vi "FPGA.Init.vi"(8 "error in (no error)":errorcluster) -> (0 "error out":errorcluster, 3 "Cluster":T1)   [LabVIEW 2015]
uses:
  Variables.ctl
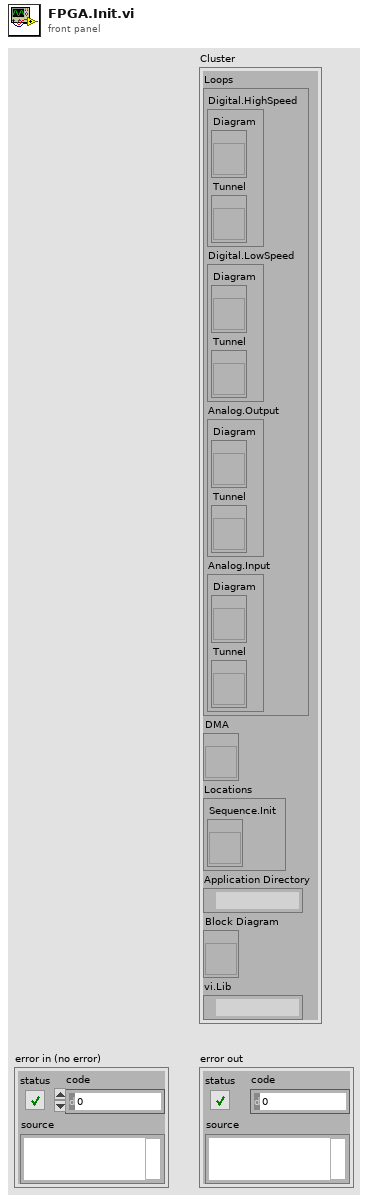
[diagram p1: front panel]
types:
  T1 = typedef "Variables.ctl" = cluster{"Loops":cluster{"Digital.HighSpeed":cluster{"Diagram":refnum<vi>, "Tunnel":refnum<vi>}, "Digital.LowSpeed":cluster{"Diagram":refnum<vi>, "Tunnel":refnum<vi>}, "Analog.Output":cluster{"Diagram":refnum<vi>, "Tunnel":refnum<vi>}, "Analog.Input":cluster{"Diagram":refnum<vi>, "Tunnel":refnum<vi>}}, "DMA":refnum<vi>, "Locations":cluster{"Sequence.Init":refnum<vi>}, "Application Directory":path, "Block Diagram":refnum<vi>, "vi.Lib":path}
  T2 = cluster{"Digital.HighSpeed":cluster{"Diagram":refnum<vi>, "Tunnel":refnum<vi>}, "Digital.LowSpeed":cluster{"Diagram":refnum<vi>, "Tunnel":refnum<vi>}, "Analog.Output":cluster{"Diagram":refnum<vi>, "Tunnel":refnum<vi>}, "Analog.Input":cluster{"Diagram":refnum<vi>, "Tunnel":refnum<vi>}}
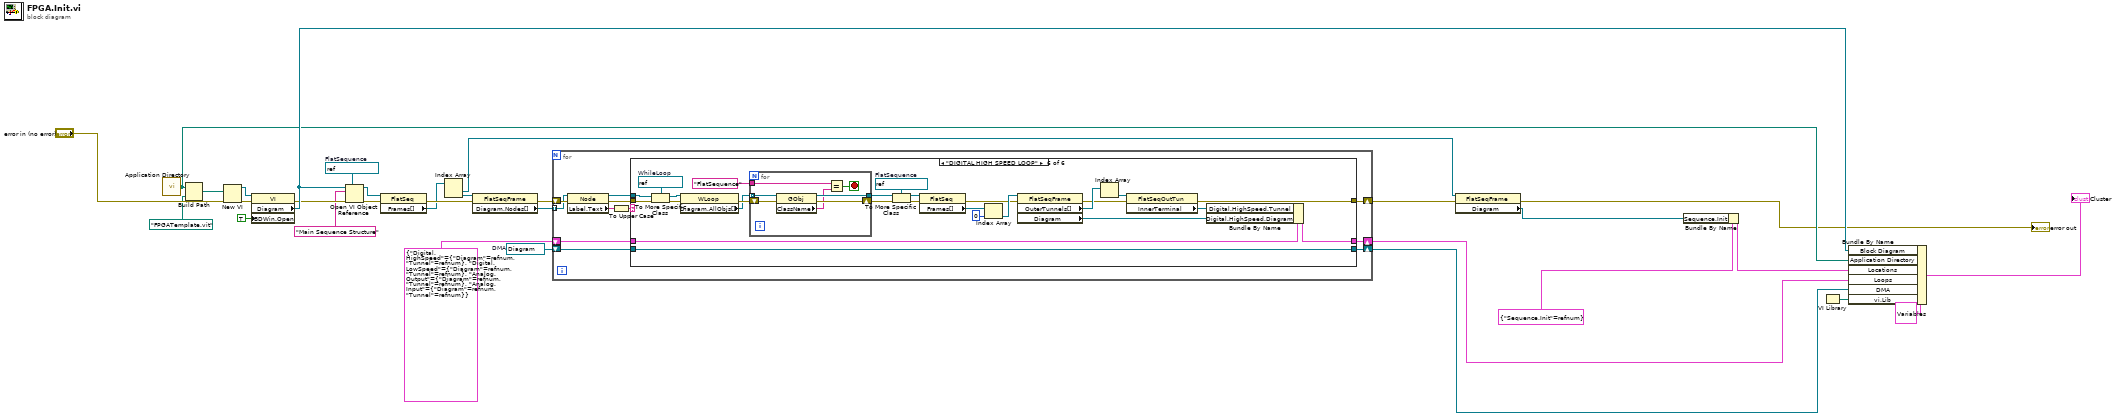
[diagram p0: block diagram]
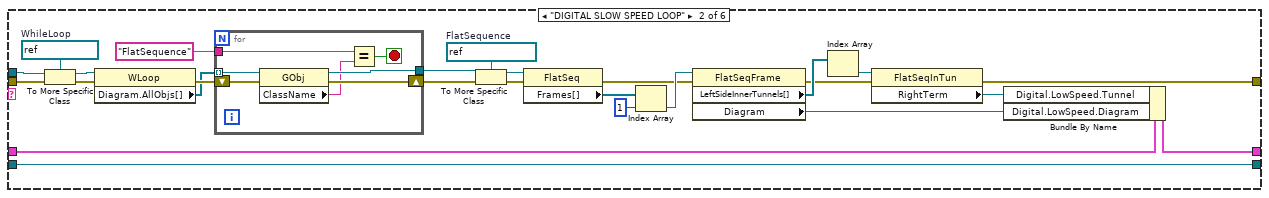
[diagram p3: hidden frame]
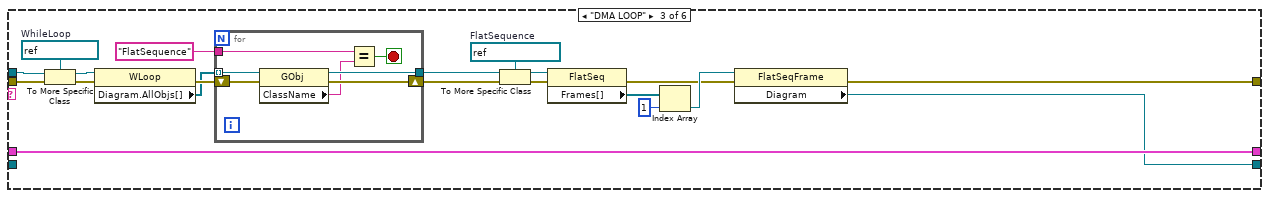
[diagram p4: hidden frame]
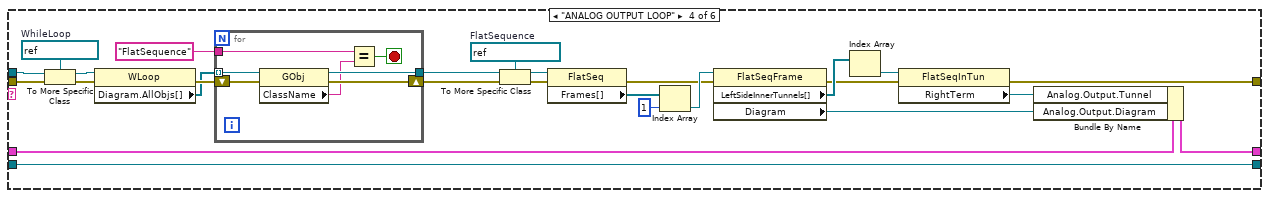
[diagram p5: hidden frame]
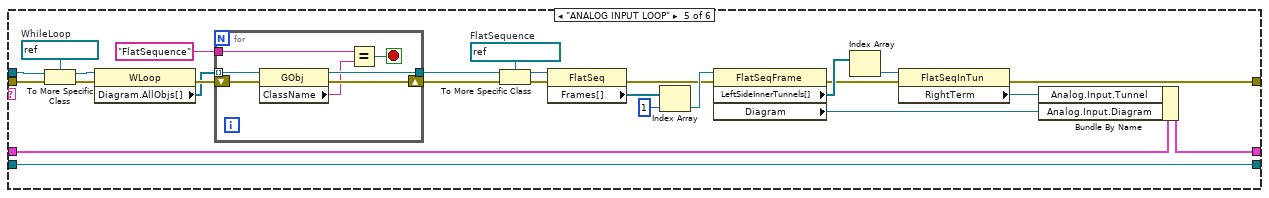
[diagram p6: hidden frame]
diagram:
  w17 = refnum<vi> refnum  # DMA
  w3 = refnum<vi> refnum  # FlatSequence
  n1 = call <vilib>:"Application Directory.vi"() -> ("Application Directory"=w28:path)
  n2 = Build Path(base path=w28, name or relative path=path "FPGATemplate.vit" ("template")) -> (appended path=w15:path)
  n3 = New VI(8:"error in (no error)", 10:w15) -> (0:w6:errorcluster, 3:w23:refnum<vi>)  [unwired: 5 in]
  n4 = property class="VI"(reference=w23, error in=w6, "BDWin.Open"=TRUE ("Block Diagram Window:Open")) -> (error out=w7:errorcluster, "Diagram"=w31:refnum<vi>)  [unwired: 1 out]
  n5 = Open VI Object Reference(7:w3, 8:w7, 10:"Main Sequence Structure" ("name/order"), 11:w31) -> (0:w9:errorcluster, 3:w8:refnum<vi>)
  n6 = property class="FlatSeq"(reference=w8, error in=w9) -> (error out=w11:errorcluster, "Frames[]"=w10:refnum<vi>[])  [unwired: 1 out]
  n7 = Index Array(array=w10) -> (element #1=w20:refnum<vi>, element #2=w18:refnum<vi>)  [unwired: 2 in]
  n8 = property class="FlatSeqFrame"(reference=w18, error in=w11) -> (error out=w13:errorcluster, "Diagram.Nodes[]"=w12:refnum<vi>[])  [unwired: 1 out]
  n9 = for {
    tunnel: w12 -> [w41] mode=indexing
    shift-right: [w35] -> w19
    shift-left: w13 -> [w42]
    shift-right: [w34] -> w27
    shift-left: T2 {"Digital.HighSpeed"={"Diagram"=refnum, "Tunnel"=refnum}, "Digital.LowSpeed"={"Diagram"=refnum, "Tunnel"=refnum}, "Analog.Output"={"Diagram"=refnum, "Tunnel"=refnum}, "Analog.Input"={"Diagram"=refnum, "Tunnel"=refnum}} -> [w38]
    shift-right: [w33] -> w30
    shift-left: w17 -> [w32]
    n10 = property class="Node"(reference=w41, error in=w42) -> (reference out=w37:refnum<vi>, error out=w36:errorcluster, "Label.Text"=w40:string)
    n11 = To Upper Case(1:w40) -> (0:w39:string)
    n12 = case shown="\"DIGITAL HIGH SPEED LOOP\"" w39 {
      tunnel: w38 -> [w44 w71 w80 w131 w164 w197]
      tunnel: w37 -> [_ w66 w95 w126 w159 w192]
      tunnel: w36 -> [w45 w67 w96 w127 w160 w193]
      tunnel: [w45 w48 w81 w107 w140 w173] -> w35
      tunnel: [w44 w70 w80 w130 w163 w196] -> w34
      tunnel: [w43 w52 w79 w112 w145 w178] -> w33
      tunnel: w32 -> [w43 w52 _ w112 w145 w178]
      frame Default {
      }
      frame "DIGITAL SLOW SPEED LOOP" {
        w65 = refnum<vi> refnum  # WhileLoop
        w58 = refnum<vi> refnum  # FlatSequence
        n13 = To More Specific Class(target class=w65, reference=w66, error in=w67) -> (specific class reference=w64:refnum<vi>, error out=w63:errorcluster)
        n14 = property class="WLoop"(reference=w64, error in=w63) -> (error out=w62:errorcluster, "Diagram.AllObjs[]"=w61:refnum<vi>[])  [unwired: 1 out]
        n15 = for {
          shift-right: [w77] -> w60
          shift-left: w62 -> [w78]
          tunnel: w61 -> [w76] mode=indexing
          tunnel: "FlatSequence" ("name/order") -> [w75]
          tunnel: [w73] -> w55
          stop <- w74 stop-if-true
          n16 = property class="GObj"(reference=w76, error in=w78) -> (reference out=w73:refnum<vi>, error out=w77:errorcluster, "ClassName"=w72:string)
          n17 = Equal?(x=w75, y=w72) -> (x = y?=w74:bool)
        }
        n18 = To More Specific Class(target class=w58, reference=w55, error in=w60) -> (specific class reference=w57:refnum<vi>, error out=w59:errorcluster)
        n19 = property class="FlatSeq"(reference=w57, error in=w59) -> (error out=w53:errorcluster, "Frames[]"=w69:refnum<vi>[])  [unwired: 1 out]
        n20 = Index Array(array=w69, index=1) -> (element=w54:refnum<vi>)
        n21 = property class="FlatSeqFrame"(reference=w54, error in=w53) -> (error out=w49:errorcluster, "LeftSideInnerTunnels[]"=w51:refnum<vi>[], "Diagram"=w46:refnum<vi>)  [unwired: 1 out]
        n22 = Index Array(array=w51) -> (element=w50:refnum<vi>)  [unwired: 1 in]
        n23 = property class="FlatSeqInTun"(reference=w50, error in=w49) -> (error out=w48:errorcluster, "RightTerm"=w47:refnum<vi>)  [unwired: 1 out]
        n24 = Bundle By Name(cluster=w71, "Digital.LowSpeed.Tunnel"=w47, "Digital.LowSpeed.Diagram"=w46) -> (w70:T2)
      }
      frame "DMA LOOP" {
        w94 = refnum<vi> refnum  # WhileLoop
        w87 = refnum<vi> refnum  # FlatSequence
        n25 = To More Specific Class(target class=w94, reference=w95, error in=w96) -> (specific class reference=w93:refnum<vi>, error out=w92:errorcluster)
        n26 = property class="WLoop"(reference=w93, error in=w92) -> (error out=w91:errorcluster, "Diagram.AllObjs[]"=w90:refnum<vi>[])  [unwired: 1 out]
        n27 = for {
          shift-right: [w104] -> w89
          shift-left: w91 -> [w105]
          tunnel: w90 -> [w103] mode=indexing
          tunnel: "FlatSequence" ("name/order") -> [w102]
          tunnel: [w100] -> w84
          stop <- w101 stop-if-true
          n28 = property class="GObj"(reference=w103, error in=w105) -> (reference out=w100:refnum<vi>, error out=w104:errorcluster, "ClassName"=w99:string)
          n29 = Equal?(x=w102, y=w99) -> (x = y?=w101:bool)
        }
        n30 = To More Specific Class(target class=w87, reference=w84, error in=w89) -> (specific class reference=w86:refnum<vi>, error out=w88:errorcluster)
        n31 = property class="FlatSeq"(reference=w86, error in=w88) -> (error out=w82:errorcluster, "Frames[]"=w98:refnum<vi>[])  [unwired: 1 out]
        n32 = Index Array(array=w98, index=1) -> (element=w83:refnum<vi>)
        n33 = property class="FlatSeqFrame"(reference=w83, error in=w82) -> (error out=w81:errorcluster, "Diagram"=w79:refnum<vi>)  [unwired: 1 out]
      }
      frame "ANALOG OUTPUT LOOP" {
        w125 = refnum<vi> refnum  # WhileLoop
        w118 = refnum<vi> refnum  # FlatSequence
        n34 = To More Specific Class(target class=w125, reference=w126, error in=w127) -> (specific class reference=w124:refnum<vi>, error out=w123:errorcluster)
        n35 = property class="WLoop"(reference=w124, error in=w123) -> (error out=w122:errorcluster, "Diagram.AllObjs[]"=w121:refnum<vi>[])  [unwired: 1 out]
        n36 = for {
          shift-right: [w137] -> w120
          shift-left: w122 -> [w138]
          tunnel: w121 -> [w136] mode=indexing
          tunnel: "FlatSequence" ("name/order") -> [w135]
          tunnel: [w133] -> w115
          stop <- w134 stop-if-true
          n37 = property class="GObj"(reference=w136, error in=w138) -> (reference out=w133:refnum<vi>, error out=w137:errorcluster, "ClassName"=w132:string)
          n38 = Equal?(x=w135, y=w132) -> (x = y?=w134:bool)
        }
        n39 = To More Specific Class(target class=w118, reference=w115, error in=w120) -> (specific class reference=w117:refnum<vi>, error out=w119:errorcluster)
        n40 = property class="FlatSeq"(reference=w117, error in=w119) -> (error out=w113:errorcluster, "Frames[]"=w129:refnum<vi>[])  [unwired: 1 out]
        n41 = Index Array(array=w129, index=1) -> (element=w114:refnum<vi>)
        n42 = property class="FlatSeqFrame"(reference=w114, error in=w113) -> (error out=w108:errorcluster, "LeftSideInnerTunnels[]"=w111:refnum<vi>[], "Diagram"=w106:refnum<vi>)  [unwired: 1 out]
        n43 = Index Array(array=w111) -> (element=w110:refnum<vi>)  [unwired: 1 in]
        n44 = property class="FlatSeqInTun"(reference=w110, error in=w108) -> (error out=w107:errorcluster, "RightTerm"=w109:refnum<vi>)  [unwired: 1 out]
        n45 = Bundle By Name(cluster=w131, "Analog.Output.Tunnel"=w109, "Analog.Output.Diagram"=w106) -> (w130:T2)
      }
      frame "ANALOG INPUT LOOP" {
        w158 = refnum<vi> refnum  # WhileLoop
        w151 = refnum<vi> refnum  # FlatSequence
        n46 = To More Specific Class(target class=w158, reference=w159, error in=w160) -> (specific class reference=w157:refnum<vi>, error out=w156:errorcluster)
        n47 = property class="WLoop"(reference=w157, error in=w156) -> (error out=w155:errorcluster, "Diagram.AllObjs[]"=w154:refnum<vi>[])  [unwired: 1 out]
        n48 = for {
          shift-right: [w170] -> w153
          shift-left: w155 -> [w171]
          tunnel: w154 -> [w169] mode=indexing
          tunnel: "FlatSequence" ("name/order") -> [w168]
          tunnel: [w166] -> w148
          stop <- w167 stop-if-true
          n49 = property class="GObj"(reference=w169, error in=w171) -> (reference out=w166:refnum<vi>, error out=w170:errorcluster, "ClassName"=w165:string)
          n50 = Equal?(x=w168, y=w165) -> (x = y?=w167:bool)
        }
        n51 = To More Specific Class(target class=w151, reference=w148, error in=w153) -> (specific class reference=w150:refnum<vi>, error out=w152:errorcluster)
        n52 = property class="FlatSeq"(reference=w150, error in=w152) -> (error out=w146:errorcluster, "Frames[]"=w162:refnum<vi>[])  [unwired: 1 out]
        n53 = Index Array(array=w162, index=1) -> (element=w147:refnum<vi>)
        n54 = property class="FlatSeqFrame"(reference=w147, error in=w146) -> (error out=w141:errorcluster, "LeftSideInnerTunnels[]"=w144:refnum<vi>[], "Diagram"=w139:refnum<vi>)  [unwired: 1 out]
        n55 = Index Array(array=w144) -> (element=w143:refnum<vi>)  [unwired: 1 in]
        n56 = property class="FlatSeqInTun"(reference=w143, error in=w141) -> (error out=w140:errorcluster, "RightTerm"=w142:refnum<vi>)  [unwired: 1 out]
        n57 = Bundle By Name(cluster=w164, "Analog.Input.Tunnel"=w142, "Analog.Input.Diagram"=w139) -> (w163:T2)
      }
      frame "DIGITAL HIGH SPEED LOOP" {
        w191 = refnum<vi> refnum  # WhileLoop
        w184 = refnum<vi> refnum  # FlatSequence
        n58 = To More Specific Class(target class=w191, reference=w192, error in=w193) -> (specific class reference=w190:refnum<vi>, error out=w189:errorcluster)
        n59 = property class="WLoop"(reference=w190, error in=w189) -> (error out=w188:errorcluster, "Diagram.AllObjs[]"=w187:refnum<vi>[])  [unwired: 1 out]
        n60 = for {
          shift-right: [w203] -> w186
          shift-left: w188 -> [w204]
          tunnel: w187 -> [w202] mode=indexing
          tunnel: "FlatSequence" ("name/order") -> [w201]
          tunnel: [w199] -> w181
          stop <- w200 stop-if-true
          n61 = property class="GObj"(reference=w202, error in=w204) -> (reference out=w199:refnum<vi>, error out=w203:errorcluster, "ClassName"=w198:string)
          n62 = Equal?(x=w201, y=w198) -> (x = y?=w200:bool)
        }
        n63 = To More Specific Class(target class=w184, reference=w181, error in=w186) -> (specific class reference=w183:refnum<vi>, error out=w185:errorcluster)
        n64 = property class="FlatSeq"(reference=w183, error in=w185) -> (error out=w179:errorcluster, "Frames[]"=w195:refnum<vi>[])  [unwired: 1 out]
        n65 = Index Array(array=w195, index=0) -> (element=w180:refnum<vi>)
        n66 = property class="FlatSeqFrame"(reference=w180, error in=w179) -> (error out=w174:errorcluster, "OuterTunnels[]"=w175:refnum<vi>[], "Diagram"=w172:refnum<vi>)  [unwired: 1 out]
        n67 = Index Array(array=w175) -> (element=w177:refnum<vi>)  [unwired: 1 in]
        n68 = property class="FlatSeqOutTun"(reference=w177, error in=w174) -> (error out=w173:errorcluster, "InnerTerminal"=w176:refnum<vi>)  [unwired: 1 out]
        n69 = Bundle By Name(cluster=w197, "Digital.HighSpeed.Tunnel"=w176, "Digital.HighSpeed.Diagram"=w172) -> (w196:T2)
      }
    }
  }
  n70 = property class="FlatSeqFrame"(reference=w20, error in=w19) -> (error out=→"error out":errorcluster, "Diagram"=w22:refnum<vi>)  [unwired: 1 out]
  n71 = Bundle By Name(cluster=cluster{"Sequence.Init":refnum<vi>} {"Sequence.Init"=refnum}, "Sequence.Init"=w22) -> (w26:cluster{"Sequence.Init":refnum<vi>})
  n72 = VI Library() -> (path=w2:path)
  n73 = Bundle By Name(cluster=T1 {"Loops"={"Digital.HighSpeed"={"Diagram"=refnum, "Tunnel"=refnum}, "Digital.LowSpeed"={"Diagram"=refnum, "Tunnel"=refnum}, "Analog.Output"={"Diagram"=refnum, "Tunnel"=refnum}, "Analog.Input"={"Diagram"=refnum, "Tunnel"=refnum}}, "DMA"=refnum, "Locations"={"Sequence.Init"=refnum}, "Application Directory"=path "", "Block Diagram"=refnum, "vi.Lib"=path ""}, "Block Diagram"=w31, "Application Directory"=w28, "Locations"=w26, "Loops"=w27, "DMA"=w30, "vi.Lib"=w2) -> (→"Cluster":T1)
